vi "update(SubVI).vi"(5 "Path":path, 6 "nim":string, 7 "Boolean":bool, 8 "error in (no error)":errorcluster, 9 "email":string, 10 "nama":string, 11 "Refnum in":T1) -> (0 "error out":errorcluster, 2 "resulting string":string, 3 "Refnum out":T1)   [LabVIEW 2024]
uses:
  <vilib>/addons/database/NI_Database_API.lvlib
  <vilib>/addons/database/Connection.llb/Conn Execute.vi
  <vilib>/addons/database/Connection.llb/Conn ObjectReference.ctl
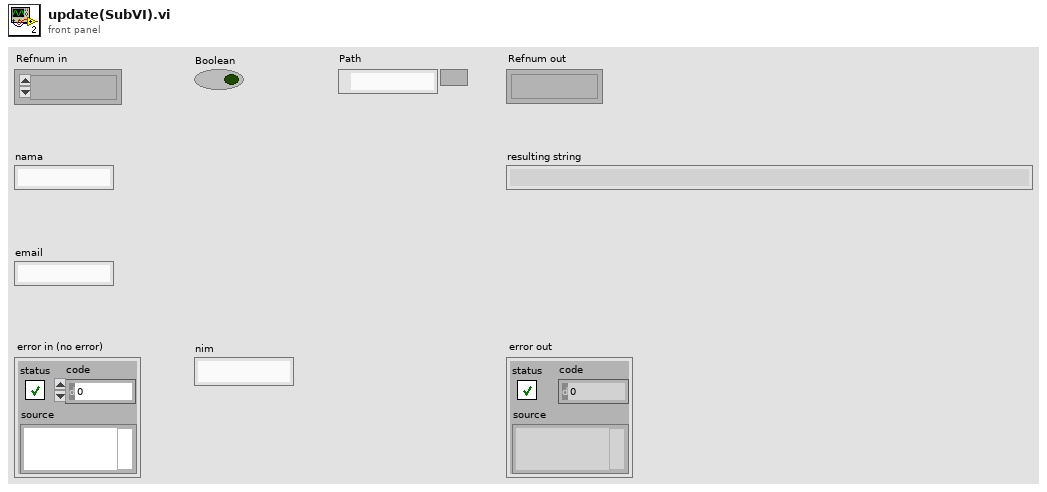
[diagram p1: front panel]
types:
  T1 = typedef "NI_Database_API.lvlib/Conn ObjectReference.ctl" = refnum<k1>
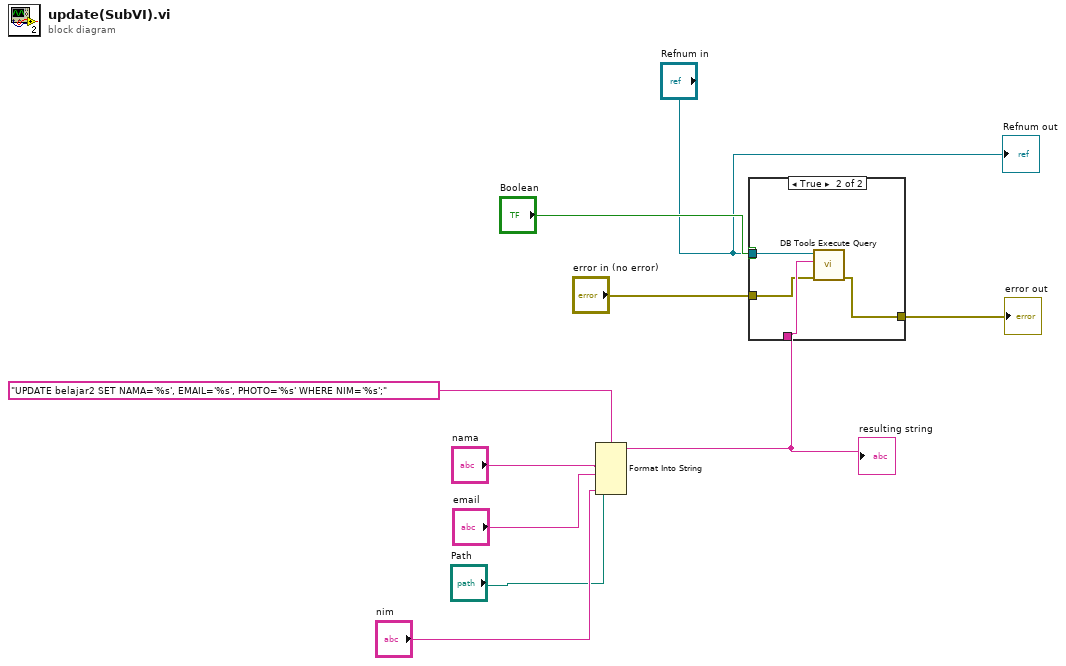
[diagram p0: block diagram]
diagram:
  n1 = Format Into String(format string="UPDATE belajar2 SET NAMA='%s', EMAIL='%s', PHOTO='%s' WHERE NIM='%s';", "nama", "email", "Path", "nim") -> (resulting string=w6:string)  [unwired: 2 in, 1 out]
  "resulting string" <- w6
  n2 = case shown="True" "Boolean" {
    tunnel: w6 -> [_ w15]
    tunnel: [w11 w14] -> w7
    tunnel: "error in (no error)" -> [w11 w13]
    tunnel: "Refnum in" -> [_ w12]
    frame False {
    }
    frame True {
      n3 = call-poly <vilib>:"DB Tools Execute Query.vi"("error in (no error)"=w13, "SQL query"=w15, "connection reference"=w12) -> ("error out"=w14:errorcluster)  [unwired: 5 in, 1 out]
    }
  }
  "error out" <- w7
  "Refnum out" <- "Refnum in"
